vi "Lab Panel V4.87.vi"() -> ()   [LabVIEW 2013] (continued)
                    n2528 = call "sub vi - cycle&temp fail v6.vi"("Amps Lo?"=w4753, "Input Cluster"=w4741, "SELECT"=w4750, "Amps Hi?"=w4749, "Result In"=w4743) -> ("(FAIL) out"=w4745:cluster{"FAIL LO":dbl, "FAIL HI":dbl}, "(DISP) out"=w4748:T4, "T-RISE"=w4742:cluster{"T-RISE (L)":dbl, "T-RISE (N)":dbl}, "Result Out"=w4744:bool, "file error"=w4747:errorcluster)  [unwired: 10 in]
                    n2529 = local write "FAIL LAB03-2"(w4745) -> ()
                    n2530 = local write "TEMP RISE LAB03-2"(w4742) -> ()
                    n2531 = local write "DISP LAB03-2"(w4748) -> ()
                    n2532 = local write "RESULT LAB03-2"(w4744) -> ()
                    n2533 = local write "data file error"(w4747) -> ()
                  }
                }
              }
              frame #6 {
                # "LAB04-1"
                n2534 = case shown="True" w4758 {
                  tunnel: w4760 -> [_ w4773]
                  tunnel: w4757 -> [_ w4770]
                  tunnel: w4759 -> [_ w4769]
                  frame False {
                  }
                  frame True {
                    n2535 = local read "TEMP START LAB04-1"() -> (w4775:cluster{"TL":dbl, "TN":dbl})
                    n2536 = local read "FAIL LAB04-1"() -> (w4766:cluster{"LO":dbl, "HI":dbl})
                    n2537 = local read "TDMS LAB04-1"() -> (w4774:refnum<k34>)
                    n2538 = local read "SET LAB04-1"() -> (w4771:T5)
                    n2539 = local read "DISP LAB04-1"() -> (w4772:T4)
                    n2540 = local read "SIG LAB04-1"() -> (w4776:T2)
                    n2541 = local read "RESULT LAB04-1"() -> (w4763:bool)
                    n2542 = Bundle("FAIL LAB04-1"=w4766, "SIG LAB04-1"=w4776, "TEMP START LAB04-1"=w4775, "DISP LAB04-1"=w4772, "SET LAB04-1"=w4771, "TDMS LAB04-1"=w4774) -> (w4761:T38)  [unwired: 1 in]
                    n2543 = call "sub vi - cycle&temp fail v6.vi"("Amps Lo?"=w4773, "Input Cluster"=w4761, "SELECT"=w4770, "Amps Hi?"=w4769, "Result In"=w4763) -> ("(FAIL) out"=w4765:cluster{"FAIL LO":dbl, "FAIL HI":dbl}, "(DISP) out"=w4768:T4, "T-RISE"=w4762:cluster{"T-RISE (L)":dbl, "T-RISE (N)":dbl}, "Result Out"=w4764:bool, "file error"=w4767:errorcluster)  [unwired: 10 in]
                    n2544 = local write "TEMP RISE LAB04-1"(w4762) -> ()
                    n2545 = local write "FAIL LAB04-1"(w4765) -> ()
                    n2546 = local write "DISP LAB04-1"(w4768) -> ()
                    n2547 = local write "RESULT LAB04-1"(w4764) -> ()
                    n2548 = local write "data file error"(w4767) -> ()
                  }
                }
              }
              frame #7 {
                # "LAB04-2"
                n2549 = case shown="True" w4778 {
                  tunnel: w4780 -> [_ w4793]
                  tunnel: w4777 -> [_ w4790]
                  tunnel: w4779 -> [_ w4789]
                  frame False {
                  }
                  frame True {
                    n2550 = local read "TEMP START LAB04-2"() -> (w4795:cluster{"TL":dbl, "TN":dbl})
                    n2551 = local read "FAIL LAB04-2"() -> (w4786:cluster{"LO":dbl, "HI":dbl})
                    n2552 = local read "TDMS LAB04-2"() -> (w4794:refnum<k34>)
                    n2553 = local read "SET LAB04-2"() -> (w4791:T5)
                    n2554 = local read "DISP LAB04-2"() -> (w4792:T4)
                    n2555 = local read "SIG LAB04-2"() -> (w4796:T2)
                    n2556 = local read "RESULT LAB04-2"() -> (w4783:bool)
                    n2557 = Bundle("FAIL LAB04-2"=w4786, "SIG LAB04-2"=w4796, "TEMP START LAB04-2"=w4795, "DISP LAB04-2"=w4792, "SET LAB04-2"=w4791, "TDMS LAB04-2"=w4794) -> (w4781:T39)  [unwired: 1 in]
                    n2558 = call "sub vi - cycle&temp fail v6.vi"("Amps Lo?"=w4793, "Input Cluster"=w4781, "SELECT"=w4790, "Amps Hi?"=w4789, "Result In"=w4783) -> ("(FAIL) out"=w4785:cluster{"FAIL LO":dbl, "FAIL HI":dbl}, "(DISP) out"=w4788:T4, "T-RISE"=w4782:cluster{"T-RISE (L)":dbl, "T-RISE (N)":dbl}, "Result Out"=w4784:bool, "file error"=w4787:errorcluster)  [unwired: 10 in]
                    n2559 = local write "TEMP RISE LAB04-2"(w4782) -> ()
                    n2560 = local write "FAIL LAB04-2"(w4785) -> ()
                    n2561 = local write "DISP LAB04-2"(w4788) -> ()
                    n2562 = local write "RESULT LAB04-2"(w4784) -> ()
                    n2563 = local write "data file error"(w4787) -> ()
                  }
                }
              }
              frame #8 {
                # "LAB05-1"
                n2564 = case shown="True" w4798 {
                  tunnel: w4800 -> [_ w4813]
                  tunnel: w4797 -> [_ w4810]
                  tunnel: w4799 -> [_ w4809]
                  frame False {
                  }
                  frame True {
                    n2565 = local read "TEMP START LAB05-1"() -> (w4815:cluster{"TL":dbl, "TN":dbl})
                    n2566 = local read "FAIL LAB05-1"() -> (w4806:cluster{"LO":dbl, "HI":dbl})
                    n2567 = local read "TDMS LAB05-1"() -> (w4814:refnum<k34>)
                    n2568 = local read "SET LAB05-1"() -> (w4811:T5)
                    n2569 = local read "DISP LAB05-1"() -> (w4812:T4)
                    n2570 = local read "SIG LAB05-1"() -> (w4816:T2)
                    n2571 = local read "RESULT LAB05-1"() -> (w4803:bool)
                    n2572 = Bundle("FAIL LAB05-1"=w4806, "SIG LAB05-1"=w4816, "TEMP START LAB05-1"=w4815, "DISP LAB05-1"=w4812, "SET LAB05-1"=w4811, "TDMS LAB05-1"=w4814) -> (w4801:T40)  [unwired: 1 in]
                    n2573 = call "sub vi - cycle&temp fail v6.vi"("Amps Lo?"=w4813, "Input Cluster"=w4801, "SELECT"=w4810, "Amps Hi?"=w4809, "Result In"=w4803) -> ("(FAIL) out"=w4805:cluster{"FAIL LO":dbl, "FAIL HI":dbl}, "(DISP) out"=w4808:T4, "T-RISE"=w4802:cluster{"T-RISE (L)":dbl, "T-RISE (N)":dbl}, "Result Out"=w4804:bool, "file error"=w4807:errorcluster)  [unwired: 10 in]
                    n2574 = local write "TEMP RISE LAB05-1"(w4802) -> ()
                    n2575 = local write "FAIL LAB05-1"(w4805) -> ()
                    n2576 = local write "DISP LAB05-1"(w4808) -> ()
                    n2577 = local write "RESULT LAB05-1"(w4804) -> ()
                    n2578 = local write "data file error"(w4807) -> ()
                  }
                }
              }
              frame #9 {
                # "LAB05-2"
                n2579 = case shown="True" w4818 {
                  tunnel: w4820 -> [_ w4833]
                  tunnel: w4817 -> [_ w4830]
                  tunnel: w4819 -> [_ w4829]
                  frame False {
                  }
                  frame True {
                    n2580 = local read "TEMP START LAB05-2"() -> (w4835:cluster{"TL":dbl, "TN":dbl})
                    n2581 = local read "FAIL LAB05-2"() -> (w4826:cluster{"LO":dbl, "HI":dbl})
                    n2582 = local read "TDMS LAB05-2"() -> (w4834:refnum<k34>)
                    n2583 = local read "SET LAB05-2"() -> (w4831:T5)
                    n2584 = local read "DISP LAB05-2"() -> (w4832:T4)
                    n2585 = local read "SIG LAB05-2"() -> (w4836:T2)
                    n2586 = local read "RESULT LAB05-2"() -> (w4823:bool)
                    n2587 = Bundle("FAIL LAB05-2"=w4826, "SIG LAB05-2"=w4836, "TEMP START LAB05-2"=w4835, "DISP LAB05-2"=w4832, "SET LAB05-2"=w4831, "TDMS LAB05-2"=w4834) -> (w4821:T41)  [unwired: 1 in]
                    n2588 = call "sub vi - cycle&temp fail v6.vi"("Amps Lo?"=w4833, "Input Cluster"=w4821, "SELECT"=w4830, "Amps Hi?"=w4829, "Result In"=w4823) -> ("(FAIL) out"=w4825:cluster{"FAIL LO":dbl, "FAIL HI":dbl}, "(DISP) out"=w4828:T4, "T-RISE"=w4822:cluster{"T-RISE (L)":dbl, "T-RISE (N)":dbl}, "Result Out"=w4824:bool, "file error"=w4827:errorcluster)  [unwired: 10 in]
                    n2589 = local write "TEMP RISE LAB05-2"(w4822) -> ()
                    n2590 = local write "FAIL LAB05-2"(w4825) -> ()
                    n2591 = local write "DISP LAB05-2"(w4828) -> ()
                    n2592 = local write "RESULT LAB05-2"(w4824) -> ()
                    n2593 = local write "data file error"(w4827) -> ()
                  }
                }
              }
            }
          }
          frame #15 {
            # "run calibration routine"
            n2594 = local read "SET (cal)"() -> (w4837:bool)
            n2595 = case shown="True" w4837 {
              frame False {
              }
              frame True {
                n2596 = stacked-sequence {
                  seq-local: [w4838 _ _] -> [_ w4840 _]
                  frame #0 {
                    n2597 = call "CALIBRATION PASSWORD"() -> ("PASSWORD"=w4838:string)  [unwired: 17 in, 2 out]
                  }
                  frame #1 {
                    n2598 = Equal?(x=w4840, y="7777") -> (x = y?=w4839:bool)
                    n2599 = case shown="True" w4839 {
                      frame False {
                      }
                      frame True {
                        n2600 = stacked-sequence {
                          frame #0 {
                            n2601 = call "sub vi - calibration v1.vi"() -> ()  [unwired: 12 in]
                          }
                          frame #1 {
                            n2602 = call "sub vi - get calibration values v1.vi"() -> ("LAB01 (CAL)"=w4846:T14, "LAB02 (CAL)"=w4845:T15, "LAB03 (CAL)"=w4844:T14, "LAB04 (CAL)"=w4843:T14, "calibration file error out"=w4847:errorcluster, "LAB05 (CAL)"=w4842:T14)  [unwired: 9 in, 1 out]
                            n2603 = local write "cal file error out"(w4847) -> ()
                            n2604 = local write "CAL LAB04"(w4843) -> ()
                            n2605 = local write "CAL LAB05"(w4842) -> ()
                            n2606 = local write "CAL LAB01"(w4846) -> ()
                            n2607 = local write "CAL LAB02"(w4845) -> ()
                            n2608 = local write "CAL LAB03"(w4844) -> ()
                          }
                        }
                      }
                    }
                  }
                  frame #2 {
                    n2609 = local write "SET (cal)"(FALSE) -> ()
                  }
                }
              }
            }
          }
          frame #16 {
            # "save certain settings to file"
            n2610 = String To Path(string="c:\\crabtree\\Set Up\\") -> (path=w4850:path)
            n2611 = Build Path(base path=w4850, name or relative path="settings.bin") -> (appended path=w4852:path)
            n2612 = Build Path(base path=w4850, name or relative path="mail.bin") -> (appended path=w4849:path)
            n2613 = Create Folder(path (use dialog)=w4850) -> (error out=w4855:errorcluster)  [unwired: 2 in, 2 out]
            n2614 = call <vilib>:"Clear Errors.vi"("error in (no error)"=w4855) -> ()  [unwired: 6 in, 1 out]
            n2615 = stacked-sequence {
              seq-local: [w4867 _] -> [_ w4880]
              tunnel: w4852 -> [_ w4881]
              tunnel: w4849 -> [_ w4879]
              frame #0 {
                n2616 = local read "C drive data root dir"() -> (w4866:path)
                n2617 = local read "Select COM port"() -> (w4863:refnum<visa-resource-name>)
                n2618 = local read "Network Directory"() -> (w4872:path)
                n2619 = local read "SET LAB05-2"() -> (w4871:T5)
                n2620 = local read "SET LAB05-1"() -> (w4870:T5)
                n2621 = local read "SET LAB04-2"() -> (w4869:T5)
                n2622 = local read "SET LAB03-2"() -> (w4873:T5)
                n2623 = local read "SET LAB04-1"() -> (w4868:T5)
                n2624 = local read "SET LAB03-1"() -> (w4874:T5)
                n2625 = local read "SET LAB02-2"() -> (w4875:T5)
                n2626 = local read "SET LAB02-1"() -> (w4876:T5)
                n2627 = local read "Temp Delay Lps"() -> (w4862:dbl)
                n2628 = local read "SET LAB01-2"() -> (w4877:T5)
                n2629 = local read "Temp Test Cal"() -> (w4859:dbl)
                n2630 = local read "SET LAB01-1"() -> (w4878:T5)
                n2631 = local read "Mail Test File To:"() -> (w4857:string)
                n2632 = local read "Temp Value"() -> (w4861:dbl)
                n2633 = local read "Fail Loops"() -> (w4860:dbl)
                n2634 = local read "spare"() -> (w4858:dbl)
                n2635 = local read "Mail Test Fail"() -> (w4856:bool)
                n2636 = local read "RATE (Hz)"() -> (w4865:dbl)
                n2637 = local read "SAMPLES"() -> (w4864:dbl)
                n2638 = Bundle("SET LAB01-1"=w4878, "SET LAB01-2"=w4877, "SET LAB02-1"=w4876, "SET LAB02-2"=w4875, "SET LAB03-1"=w4874, "SET LAB03-2"=w4873, "SET LAB04-1"=w4868, "SET LAB04-2"=w4869, "SET LAB05-1"=w4870, "SET LAB05-2"=w4871, "Network Directory"=w4872, "C drive data root dir"=w4866, "RATE (Hz)"=w4865, "SAMPLES"=w4864, "Select COM port"=w4863, "Temp Delay Lps"=w4862, "Temp Value"=w4861, "Fail Loops"=w4860, "Temp Test Cal"=w4859, "spare"=w4858, "Mail Test File To:"=w4857, "Mail Test Fail"=w4856) -> (w4867:T22)  [unwired: 1 in]
              }
              frame #1 {
                n2639 = event shown="[1] \"SET LAB01-1\", \"SET LAB01-2\", \"SET LAB02-1\", \"SET LAB02-2\", \"SET LAB03-1\", \"SET LAB03-2\", \"SET LAB04-1\", \"SET LAB04-2\", \"SET LAB05-1\", \"SET LAB05-2\", \"Network Directory\", \"C drive data root dir\", \"RATE (Hz)\", \"SAMPLES\", \"Select COM port\", \"Temp Delay Lps\", \"Temp Value\", \"Fail Loops\", \"Temp Test Cal\", \"spare\", \"Mail Test File To:\", \"Mail Test Fail\": Value Change" {
                  selector: _ -> [_ _ _]
                  dyn-events: _ -> [_ _ _]
                  timeout: 10.0 -> [_ _ _]
                  tunnel: w4881 -> [_ w4883 _]
                  tunnel: w4880 -> [_ w4884 _]
                  tunnel: w4879 -> [_ _ w4895]
                  event Timeout {
                    n2640 = event-data() -> ()  [unwired: 1 in, 3 out]
                  }
                  event "SET LAB01-1", "SET LAB01-2", "SET LAB02-1", "SET LAB02-2", "SET LAB03-1", "SET LAB03-2", "SET LAB04-1", "SET LAB04-2", "SET LAB05-1", "SET LAB05-2", "Network Directory", "C drive data root dir", "RATE (Hz)", "SAMPLES", "Select COM port", "Temp Delay Lps", "Temp Value", "Fail Loops", "Temp Test Cal", "spare", "Mail Test File To:", "Mail Test Fail": Value Change {
                    n2641 = event-data() -> ()  [unwired: 1 in, 6 out]
                    n2642 = Open/Create/Replace File(file path (use dialog)=w4883, operation (0:open)=T21."replace or create") -> (refnum out=w4889:refnum<file>, error out=w4888:errorcluster)  [unwired: 4 in, 1 out]
                    n2643 = Write to Binary File(file (use dialog)=w4889, data=w4884, error in=w4888) -> (refnum out=w4887:refnum<file>, error out=w4886:errorcluster)  [unwired: 3 in, 1 out]
                    n2644 = Close File(refnum=w4887, error in=w4886) -> (error out=w4885:errorcluster)  [unwired: 1 out]
                    n2645 = local write "data file error"(w4885) -> ()
                  }
                  event "MAIL SETTINGS.OUT SERVER ADDRESS", "MAIL SETTINGS.FROM ACCOUNT", "MAIL SETTINGS.USER NAME", "MAIL SETTINGS.PASSWORD", "Auto Mail Send", "TO (string):": Value Change {
                    n2646 = event-data() -> ()  [unwired: 1 in, 6 out]
                    n2647 = local read "MAIL SETTINGS"() -> (w4894:T7)
                    n2648 = local read "Auto Mail Send"() -> (w4892:bool)
                    n2649 = local read "TO (string):"() -> (w4891:string)
                    n2650 = Open/Create/Replace File(file path (use dialog)=w4895, operation (0:open)=T21."replace or create") -> (refnum out=w4900:refnum<file>, error out=w4899:errorcluster)  [unwired: 4 in, 1 out]
                    n2651 = Bundle("MAIL SETTINGS"=w4894, "Auto Mail Send"=w4892, "TO (string):"=w4891) -> (w4893:T42)  [unwired: 1 in]
                    n2652 = Write to Binary File(file (use dialog)=w4900, data=w4893, error in=w4899) -> (refnum out=w4898:refnum<file>, error out=w4897:errorcluster)  [unwired: 3 in, 1 out]
                    n2653 = Close File(refnum=w4898, error in=w4897) -> (error out=w4896:errorcluster)  [unwired: 1 out]
                    n2654 = local write "data file error"(w4896) -> ()
                  }
                }
              }
            }
          }
          frame #17 {
            # "mail control"
            n2655 = local read "MAIL SETTINGS"() -> (w4917:T7)
            n2656 = local read "Auto Mail Send"() -> (w4903:bool)
            n2657 = Unbundle(w4917) -> ("OUT SERVER ADDRESS"=w4916:string, "FROM ACCOUNT"=w4915:string, "TEST MAIL"=w4914:bool)  [unwired: 4 out]
            n2658 = stacked-sequence {
              tunnel: "TO (string):" -> [_ w4956]
              tunnel: w4917 -> [w4922 w4955]
              tunnel: w4916 -> [w4921 w4954]
              tunnel: w4915 -> [w4920 w4953]
              tunnel: w4914 -> [w4919 _]
              tunnel: w4903 -> [_ w4952]
              tunnel: w4913 -> [_ w4951]
              tunnel: w4912 -> [_ w4950]
              tunnel: w4911 -> [_ w4949]
              tunnel: w4910 -> [_ w4948]
              tunnel: w4909 -> [_ w4947]
              tunnel: w4908 -> [_ w4946]
              tunnel: w4907 -> [_ w4945]
              tunnel: w4906 -> [_ w4944]
              tunnel: w4905 -> [_ w4943]
              tunnel: w4904 -> [_ w4942]
              tunnel: "TO (string):" -> [w4918 _]
              frame #0 {
                # "mail test"
                n2659 = case shown="True" w4919 {
                  tunnel: w4922 -> [_ w4926]
                  tunnel: w4918 -> [_ w4925]
                  tunnel: w4921 -> [_ w4924]
                  tunnel: w4920 -> [_ w4923]
                  frame False {
                  }
                  frame True {
                    n2660 = stacked-sequence {
                      seq-local: [_ _ w4936 _] -> [_ _ _ w4937]
                      tunnel: w4926 -> [w4929 _ _ w4941]
                      tunnel: w4925 -> [_ _ w4934 _]
                      tunnel: w4924 -> [_ _ w4932 _]
                      tunnel: w4923 -> [_ _ w4933 _]
                      frame #0 {
                        n2661 = Bundle(cluster=w4929, "TEST MAIL STATUS"="TEST START") -> (w4927:T7)  [unwired: 6 in]
                        n2662 = local write "MAIL SETTINGS"(w4927) -> ()
                      }
                      frame #1 {
                        n2663 = Wait (ms)(milliseconds to wait=500) -> ()  [unwired: 1 out]
                      }
                      frame #2 {
                        n2664 = call "sub vi - send mail v5.vi"("TO:"=w4934, "subject"="MAIL TEST FROM LAB PANEL", "from"=w4933, "out going server"=w4932, "message"="TEST MESSAGE") -> ("error out"=w4936:errorcluster)  [unwired: 10 in]
                      }
                      frame #3 {
                        n2665 = Bundle(cluster=w4941, "TEST MAIL"=FALSE, "TEST MAIL STATUS"="TEST END", "mail error"=w4937) -> (w4939:T7)  [unwired: 4 in]
                        n2666 = local write "MAIL SETTINGS"(w4939) -> ()
                      }
                    }
                  }
                }
              }
              frame #1 {
                # "mail report"
                n2667 = stacked-sequence {
                  seq-local: [_ w4999 _ _] -> [_ _ _ w5189]
                  seq-local: [_ _ w5102 _] -> [_ _ _ w5179]
                  seq-local: [w4966 _ _ _] -> [_ w5016 _ _]
                  seq-local: [w4965 _ _ _] -> [_ w5015 _ _]
                  seq-local: [w4963 _ _ _] -> [_ w5013 _ _]
                  seq-local: [w4964 _ _ _] -> [_ w5014 _ _]
                  seq-local: [w4962 _ _ _] -> [_ w5012 _ _]
                  seq-local: [w4961 _ _ _] -> [_ w5007 _ _]
                  seq-local: [w4960 _ _ _] -> [_ w5008 _ _]
                  seq-local: [w4959 _ _ _] -> [_ w5009 _ _]
                  seq-local: [w4958 _ _ _] -> [_ w5010 _ _]
                  seq-local: [w4957 _ _ _] -> [_ w5011 _ _]
                  tunnel: w4956 -> [_ _ _ w5190]
                  tunnel: w4955 -> [_ _ _ w5173]
                  tunnel: w4954 -> [_ _ _ w5187]
                  tunnel: w4953 -> [_ _ _ w5186]
                  tunnel: w4952 -> [w4997 _ _ w5181]
                  tunnel: w4951 -> [_ _ w5132 _]
                  tunnel: w4950 -> [_ _ w5129 _]
                  tunnel: w4949 -> [_ _ w5128 _]
                  tunnel: w4948 -> [_ _ w5127 _]
                  tunnel: w4947 -> [_ _ w5126 _]
                  tunnel: w4946 -> [_ _ w5125 _]
                  tunnel: w4945 -> [_ _ w5124 _]
                  tunnel: w4944 -> [_ _ w5123 _]
                  tunnel: w4943 -> [_ _ w5122 _]
                  tunnel: w4942 -> [_ _ w5121 _]
                  frame #0 {
                    n2668 = case shown="False" w4997 {
                      frame False {
                        n2669 = local write "mail control"("") -> ()
                      }
                      frame True {
                      }
                    }
                    n2670 = local read "SET LAB01-1"() -> (w4996:T5)
                    n2671 = local read "SET LAB01-2"() -> (w4995:T5)
                    n2672 = local read "SET LAB02-1"() -> (w4994:T5)
                    n2673 = local read "SET LAB02-2"() -> (w4993:T5)
                    n2674 = local read "SET LAB03-1"() -> (w4992:T5)
                    n2675 = local read "SET LAB04-1"() -> (w4990:T5)
                    n2676 = local read "SET LAB05-1"() -> (w4988:T5)
                    n2677 = local read "SET LAB03-2"() -> (w4991:T5)
                    n2678 = local read "SET LAB04-2"() -> (w4989:T5)
                    n2679 = local read "SET LAB05-2"() -> (w4987:T5)
                    n2680 = Unbundle(w4992) -> ("DESCRIPTION"=w4972:string)  [unwired: 4 out]
                    n2681 = Unbundle(w4991) -> ("DESCRIPTION"=w4971:string)  [unwired: 4 out]
                    n2682 = Unbundle(w4990) -> ("DESCRIPTION"=w4970:string)  [unwired: 4 out]
                    n2683 = Unbundle(w4987) -> ("DESCRIPTION"=w4967:string)  [unwired: 4 out]
                    n2684 = Unbundle(w4993) -> ("DESCRIPTION"=w4973:string)  [unwired: 4 out]
                    n2685 = Unbundle(w4989) -> ("DESCRIPTION"=w4969:string)  [unwired: 4 out]
                    n2686 = Unbundle(w4996) -> ("DESCRIPTION"=w4985:string)  [unwired: 4 out]
                    n2687 = Unbundle(w4994) -> ("DESCRIPTION"=w4974:string)  [unwired: 4 out]
                    n2688 = Unbundle(w4988) -> ("DESCRIPTION"=w4968:string)  [unwired: 4 out]
                    n2689 = Unbundle(w4995) -> ("DESCRIPTION"=w4975:string)  [unwired: 4 out]
                    n2690 = Concatenate Strings("[LAB05-2/", w4967) -> (w4957:string)
                    n2691 = Concatenate Strings("[LAB05-1/", w4968) -> (w4958:string)
                    n2692 = Concatenate Strings("[LAB04-2/", w4969) -> (w4959:string)
                    n2693 = Concatenate Strings("[LAB03-2/", w4971) -> (w4961:string)
                    n2694 = Concatenate Strings("[LAB04-1/", w4970) -> (w4960:string)
                    n2695 = Concatenate Strings("[LAB03-1/", w4972) -> (w4962:string)
                    n2696 = Concatenate Strings("[LAB01-2/", w4975) -> (w4965:string)
                    n2697 = Concatenate Strings("[LAB02-2/", w4973) -> (w4963:string)
                    n2698 = Concatenate Strings("[LAB01-1/", w4985) -> (w4966:string)
                    n2699 = Concatenate Strings("[LAB02-1/", w4974) -> (w4964:string)
                  }
                  frame #1 {
                    w5020 = "/"
                    w5021 = 2.0
                    n2700 = local read "DISP LAB01-2"() -> (w5100:T4)
                    n2701 = local read "DISP LAB01-1"() -> (w5101:T4)
                    n2702 = local read "DISP LAB02-1"() -> (w5099:T4)
                    n2703 = local read "DISP LAB03-2"() -> (w5096:T4)
                    n2704 = local read "DISP LAB02-2"() -> (w5098:T4)
                    n2705 = local read "DISP LAB03-1"() -> (w5097:T4)
                    n2706 = local read "DISP LAB04-2"() -> (w5094:T4)
                    n2707 = local read "DISP LAB04-1"() -> (w5095:T4)
                    n2708 = local read "DISP LAB05-1"() -> (w5093:T4)
                    n2709 = local read "DISP LAB05-2"() -> (w5092:T4)
                    n2710 = Unbundle(w5100) -> ("CYCLE"=w5084:dbl, "MINS"=w5083:dbl, "STATUS"=w5080:string)
                    n2711 = Unbundle(w5101) -> ("CYCLE"=w5089:dbl, "MINS"=w5088:dbl, "STATUS"=w5085:string)
                    n2712 = Unbundle(w5099) -> ("CYCLE"=w5077:dbl, "MINS"=w5076:dbl, "STATUS"=w5075:string)
                    n2713 = Unbundle(w5096) -> ("CYCLE"=w5064:dbl, "MINS"=w5063:dbl, "STATUS"=w5060:string)
                    n2714 = Unbundle(w5097) -> ("CYCLE"=w5069:dbl, "MINS"=w5068:dbl, "STATUS"=w5065:string)
                    n2715 = Unbundle(w5098) -> ("CYCLE"=w5074:dbl, "MINS"=w5073:dbl, "STATUS"=w5070:string)
                    n2716 = Unbundle(w5095) -> ("CYCLE"=w5059:dbl, "MINS"=w5058:dbl, "STATUS"=w5055:string)
                    n2717 = Unbundle(w5094) -> ("CYCLE"=w5054:dbl, "MINS"=w5053:dbl, "STATUS"=w5050:string)
                    n2718 = Unbundle(w5093) -> ("CYCLE"=w5049:dbl, "MINS"=w5048:dbl, "STATUS"=w5045:string)
                    n2719 = Unbundle(w5092) -> ("CYCLE"=w5091:dbl, "MINS"=w5090:dbl, "STATUS"=w5042:string)
                    n2720 = Number To Decimal String(number=w5077) -> (decimal integer string=w5079:string)  [unwired: 1 in]
                    n2721 = Number To Decimal String(number=w5074) -> (decimal integer string=w5072:string)  [unwired: 1 in]
                    n2722 = Number To Decimal String(number=w5069) -> (decimal integer string=w5067:string)  [unwired: 1 in]
                    n2723 = Number To Decimal String(number=w5084) -> (decimal integer string=w5082:string)  [unwired: 1 in]
                    n2724 = Number To Decimal String(number=w5064) -> (decimal integer string=w5062:string)  [unwired: 1 in]
                    n2725 = Number To Decimal String(number=w5089) -> (decimal integer string=w5087:string)  [unwired: 1 in]
                    n2726 = Number To Decimal String(number=w5091) -> (decimal integer string=w5044:string)  [unwired: 1 in]
                    n2727 = Number To Decimal String(number=w5059) -> (decimal integer string=w5057:string)  [unwired: 1 in]
                    n2728 = Number To Decimal String(number=w5054) -> (decimal integer string=w5052:string)  [unwired: 1 in]
                    n2729 = Number To Decimal String(number=w5049) -> (decimal integer string=w5047:string)  [unwired: 1 in]
                    n2730 = Number To Fractional String(number=w5076, precision (6)=w5021) -> (F-format string=w5078:string)  [unwired: 2 in]
                    n2731 = Number To Fractional String(number=w5063, precision (6)=w5021) -> (F-format string=w5061:string)  [unwired: 2 in]
                    n2732 = Number To Fractional String(number=w5073, precision (6)=w5021) -> (F-format string=w5071:string)  [unwired: 2 in]
                    n2733 = Number To Fractional String(number=w5068, precision (6)=w5021) -> (F-format string=w5066:string)  [unwired: 2 in]
                    n2734 = Number To Fractional String(number=w5053, precision (6)=w5021) -> (F-format string=w5051:string)  [unwired: 2 in]
                    n2735 = Number To Fractional String(number=w5058, precision (6)=w5021) -> (F-format string=w5056:string)  [unwired: 2 in]
                    n2736 = Number To Fractional String(number=w5083, precision (6)=w5021) -> (F-format string=w5081:string)  [unwired: 2 in]
                    n2737 = Number To Fractional String(number=w5048, precision (6)=w5021) -> (F-format string=w5046:string)  [unwired: 2 in]
                    n2738 = Number To Fractional String(number=w5088, precision (6)=w5021) -> (F-format string=w5086:string)  [unwired: 2 in]
                    n2739 = Number To Fractional String(number=w5090, precision (6)=w5021) -> (F-format string=w5043:string)  [unwired: 2 in]
                    n2740 = Concatenate Strings(w5020, w5062, w5020, w5061, w5020, w5060) -> (w5036:string)
                    n2741 = Concatenate Strings(w5020, w5057, w5020, w5056, w5020, w5055) -> (w5035:string)
                    n2742 = Concatenate Strings(w5020, w5052, w5020, w5051, w5020, w5050) -> (w5034:string)
                    n2743 = Concatenate Strings(w5020, w5047, w5020, w5046, w5020, w5045) -> (w5033:string)
                    n2744 = Concatenate Strings(w5020, w5044, w5020, w5043, w5020, w5042) -> (w5032:string)
                    n2745 = Concatenate Strings(w5020, w5087, w5020, w5086, w5020, w5085) -> (w5041:string)
                    n2746 = Concatenate Strings(w5020, w5067, w5020, w5066, w5020, w5065) -> (w5037:string)
                    n2747 = Concatenate Strings(w5020, w5082, w5020, w5081, w5020, w5080) -> (w5040:string)
                    n2748 = Concatenate Strings(w5020, w5079, w5020, w5078, w5020, w5075) -> (w5039:string)
                    n2749 = Concatenate Strings(w5020, w5072, w5020, w5071, w5020, w5070) -> (w5038:string)
                    n2750 = Concatenate Strings("]", "\r") -> (w5017:string)
                    n2751 = Concatenate Strings(w5012, w5037, w5017) -> (w5027:string)
                    n2752 = Concatenate Strings(w5014, w5039, w5017) -> (w5029:string)
                    n2753 = Concatenate Strings(w5013, w5038, w5017) -> (w5028:string)
                    n2754 = Concatenate Strings(w5009, w5034, w5017) -> (w5024:string)
                    n2755 = Concatenate Strings(w5010, w5033, w5017) -> (w5025:string)
                    n2756 = Concatenate Strings(w5008, w5035, w5017) -> (w5023:string)
                    n2757 = Concatenate Strings(w5007, w5036, w5017) -> (w5022:string)
                    n2758 = Concatenate Strings(w5011, w5032, w5017) -> (w5026:string)
                    n2759 = Concatenate Strings(w5015, w5040, w5017) -> (w5030:string)
                    n2760 = Concatenate Strings(w5016, w5041, w5017) -> (w5031:string)
                    n2761 = Concatenate Strings(w5031, w5030, w5029, w5028, w5027, w5022, w5023, w5024, w5025, w5026) -> (w5000:string)
                    n2762 = Concatenate Strings("[PANEL/", "DESC/", "CYCLES/", "MINS/", "STATUS]", "\r", w5000) -> (w4999:string)
                    "MAIL REPORT" <- w4999
                    n2763 = global write "Global display 3.vi" "log all"(w4999) -> ()
                  }
                  frame #2 {
                    w5130 = "END"
                    n2764 = local read "mail control"() -> (w5131:string)
                    n2765 = case shown="False" w5126 {
                      tunnel: w5131 -> [w5155 _]
                      tunnel: w5130 -> [w5154 _]
                      tunnel: [w5153 FALSE] -> w5116
                      frame False {
                        n2766 = Equal?(x=w5155, y=w5154) -> (x = y?=w5153:bool)
                      }
                      frame True {
                      }
                    }
                    n2767 = case shown="False" w5132 {
                      tunnel: w5131 -> [w5171 _]
                      tunnel: w5130 -> [w5170 _]
                      tunnel: [w5169 FALSE] -> w5120
                      frame False {
                        n2768 = Equal?(x=w5171, y=w5170) -> (x = y?=w5169:bool)
                      }
                      frame True {
                      }
                    }
                    n2769 = case shown="False" w5129 {
                      tunnel: w5131 -> [w5167 _]
                      tunnel: w5130 -> [w5166 _]
                      tunnel: [w5165 FALSE] -> w5119
                      frame False {
                        n2770 = Equal?(x=w5167, y=w5166) -> (x = y?=w5165:bool)
                      }
                      frame True {
                      }
                    }
                    n2771 = case shown="False" w5127 {
                      tunnel: w5131 -> [w5159 _]
                      tunnel: w5130 -> [w5158 _]
                      tunnel: [w5157 FALSE] -> w5117
                      frame False {
                        n2772 = Equal?(x=w5159, y=w5158) -> (x = y?=w5157:bool)
                      }
                      frame True {
                      }
                    }
                    n2773 = case shown="False" w5128 {
                      tunnel: w5131 -> [w5163 _]
                      tunnel: w5130 -> [w5162 _]
                      tunnel: [w5161 FALSE] -> w5118
                      frame False {
                        n2774 = Equal?(x=w5163, y=w5162) -> (x = y?=w5161:bool)
                      }
                      frame True {
                      }
                    }
                    n2775 = Or(x=w5118, y=w5117) -> (x .or. y?=w5109:bool)
                    n2776 = Or(x=w5120, y=w5119) -> (x .or. y?=w5110:bool)
                    n2777 = Or(x=w5110, y=w5109) -> (x .or. y?=w5105:bool)
                    n2778 = case shown="False" w5122 {
                      tunnel: w5131 -> [w5139 _]
                      tunnel: w5130 -> [w5138 _]
                      tunnel: [w5137 FALSE] -> w5111
                      frame False {
                        n2779 = Equal?(x=w5139, y=w5138) -> (x = y?=w5137:bool)
                      }
                      frame True {
                      }
                    }
                    n2780 = case shown="False" w5121 {
                      tunnel: w5131 -> [w5135 _]
                      tunnel: w5130 -> [w5134 _]
                      tunnel: [w5133 FALSE] -> w5115
                      frame False {
                        n2781 = Equal?(x=w5135, y=w5134) -> (x = y?=w5133:bool)
                      }
                      frame True {
                      }
                    }
                    n2782 = case shown="False" w5123 {
                      tunnel: w5131 -> [w5143 _]
                      tunnel: w5130 -> [w5142 _]
                      tunnel: [w5141 FALSE] -> w5112
                      frame False {
                        n2783 = Equal?(x=w5143, y=w5142) -> (x = y?=w5141:bool)
                      }
                      frame True {
                      }
                    }
                    n2784 = case shown="False" w5125 {
                      tunnel: w5131 -> [w5151 _]
                      tunnel: w5130 -> [w5150 _]
                      tunnel: [w5149 FALSE] -> w5114
                      frame False {
                        n2785 = Equal?(x=w5151, y=w5150) -> (x = y?=w5149:bool)
                      }
                      frame True {
                      }
                    }
                    n2786 = case shown="False" w5124 {
                      tunnel: w5131 -> [w5147 _]
                      tunnel: w5130 -> [w5146 _]
                      tunnel: [w5145 FALSE] -> w5113
                      frame False {
                        n2787 = Equal?(x=w5147, y=w5146) -> (x = y?=w5145:bool)
                      }
                      frame True {
                      }
                    }
                    n2788 = Or(x=w5114, y=w5113) -> (x .or. y?=w5108:bool)
                    n2789 = Or(x=w5112, y=w5111) -> (x .or. y?=w5107:bool)
                    n2790 = Or(x=w5115, y=w5116) -> (x .or. y?=w5103:bool)
                    n2791 = Or(x=w5108, y=w5107) -> (x .or. y?=w5106:bool)
                    n2792 = Or(x=w5105, y=w5106) -> (x .or. y?=w5104:bool)
                    n2793 = Or(x=w5104, y=w5103) -> (x .or. y?=w5102:bool)
                  }
                  frame #3 {
                    n2794 = local read "on loops"() -> (w5185:dbl)
                    n2795 = local read "jig cycle"() -> (w5182:dbl)
                    n2796 = local read "Send Mail Now"() -> (w5176:bool)
                    n2797 = Add(x=w5185, y=3.0) -> (x+y=w5183:dbl)
                    n2798 = Equal?(x=w5182, y=w5183) -> (x = y?=w5177:bool)
                    n2799 = And(x=w5177, y=w5176) -> (x .and. y?=w5175:bool)
                    n2800 = And(x=w5181, y=w5177) -> (x .and. y?=w5180:bool)
                    n2801 = And(x=w5180, y=w5179) -> (x .and. y?=w5178:bool)
                    n2802 = Or(x=w5178, y=w5175) -> (x .or. y?=w5174:bool)
                    n2803 = case shown="True" w5174 {
                      tunnel: w5190 -> [_ w5196]
                      tunnel: w5189 -> [_ w5195]
                      tunnel: "Lab Panel Test Status" -> [_ w5194]
                      tunnel: w5187 -> [_ w5193]
                      tunnel: w5186 -> [_ w5192]
                      tunnel: w5173 -> [_ w5191]
                      frame False {
                      }
                      frame True {
                        n2804 = stacked-sequence {
                          tunnel: w5196 -> [w5204 _]
                          tunnel: w5195 -> [w5203 _]
                          tunnel: w5194 -> [w5202 _]
                          tunnel: w5193 -> [w5201 _]
                          tunnel: w5192 -> [w5200 _]
                          tunnel: w5191 -> [w5199 _]
                          frame #0 {
                            n2805 = call "sub vi - send mail v5.vi"("TO:"=w5204, "subject"=w5202, "from"=w5200, "out going server"=w5201, "message"=w5203) -> ("error out"=w5198:errorcluster)  [unwired: 10 in]
                            n2806 = Bundle(cluster=w5199, "mail error"=w5198) -> (w5197:T7)  [unwired: 6 in]
                            n2807 = local write "MAIL SETTINGS"(w5197) -> ()
                          }
                          frame #1 {
                            n2808 = local write "mail control"("") -> ()
                            n2809 = local write "Send Mail Now"(FALSE) -> ()
                          }
                        }
                      }
                    }
                  }
                }
              }
            }
          }
          frame #18 {
            # "save jig cycle values once all run switches are off"
            n2810 = stacked-sequence {
              tunnel: w5216 -> [_ w5245]
              tunnel: w5215 -> [_ w5244]
              tunnel: w5214 -> [_ w5243]
              tunnel: w5213 -> [_ w5242]
              tunnel: w5212 -> [_ w5241]
              tunnel: w5211 -> [_ w5240]
              tunnel: w5210 -> [_ w5239]
              tunnel: w5209 -> [_ w5238]
              tunnel: w5208 -> [_ w5237]
              tunnel: w5207 -> [_ w5236]
              frame #0 {
              }
              frame #1 {
                n2811 = Not(x=w5236) -> (.not. x?=w5219:bool)
                n2812 = Not(x=w5244) -> (.not. x?=w5234:bool)
                n2813 = Not(x=w5241) -> (.not. x?=w5229:bool)
                n2814 = Not(x=w5239) -> (.not. x?=w5225:bool)
                n2815 = Not(x=w5237) -> (.not. x?=w5221:bool)
                n2816 = Not(x=w5245) -> (.not. x?=w5235:bool)
                n2817 = Not(x=w5243) -> (.not. x?=w5233:bool)
                n2818 = Not(x=w5240) -> (.not. x?=w5227:bool)
                n2819 = Not(x=w5242) -> (.not. x?=w5231:bool)
                n2820 = Not(x=w5238) -> (.not. x?=w5223:bool)
                n2821 = local read "Save JC"() -> (w5247:bool)
                n2822 = And(x=w5235, y=w5234) -> (x .and. y?=w5232:bool)
                n2823 = And(x=w5232, y=w5233) -> (x .and. y?=w5230:bool)
                n2824 = And(x=w5230, y=w5231) -> (x .and. y?=w5228:bool)
                n2825 = And(x=w5228, y=w5229) -> (x .and. y?=w5226:bool)
                n2826 = And(x=w5226, y=w5227) -> (x .and. y?=w5224:bool)
                n2827 = And(x=w5224, y=w5225) -> (x .and. y?=w5222:bool)
                n2828 = And(x=w5222, y=w5223) -> (x .and. y?=w5220:bool)
                n2829 = And(x=w5220, y=w5221) -> (x .and. y?=w5218:bool)
                n2830 = And(x=w5218, y=w5219) -> (x .and. y?=w5217:bool)
                n2831 = And(x=w5217, y=w5247) -> (x .and. y?=w5246:bool)
                n2832 = case shown="True" w5246 {
                  tunnel: w5217 -> [w5248 _]
                  frame False {
                    n2833 = case shown="False" w5248 {
                      frame False {
                        n2834 = local write "Save JC"(TRUE) -> ()
                      }
                      frame True {
                      }
                    }
                  }
                  frame True {
                    n2835 = stacked-sequence {
                      frame #0 {
                        n2836 = String To Path(string="c:\\crabtree\\Jig Cycles\\") -> (path=w5260:path)
                        n2837 = Build Path(base path=w5260, name or relative path="jigcycles.bin") -> (appended path=w5258:path)
                        n2838 = Create Folder(path (use dialog)=w5260) -> (error out=w5262:errorcluster)  [unwired: 2 in, 2 out]
                        n2839 = local read "JIG RELAY CYCLES"() -> (w5252:T8)
                        n2840 = call <vilib>:"Clear Errors.vi"("error in (no error)"=w5262) -> ()  [unwired: 6 in, 1 out]
                        n2841 = local write "Save JC"(FALSE) -> ()
                        n2842 = Open/Create/Replace File(file path (use dialog)=w5258, operation (0:open)=T21."replace or create") -> (refnum out=w5256:refnum<file>, error out=w5257:errorcluster)  [unwired: 4 in, 1 out]
                        n2843 = Write to Binary File(file (use dialog)=w5256, data=w5252, error in=w5257) -> (refnum out=w5255:refnum<file>, error out=w5254:errorcluster)  [unwired: 3 in, 1 out]
                        n2844 = Close File(refnum=w5255, error in=w5254) -> (error out=w5253:errorcluster)  [unwired: 1 out]
                        n2845 = local write "data file error"(w5253) -> ()
                      }
                      frame #1 {
                        n2846 = local read "JIG RELAY CYCLES"() -> (w5285:T8)
                        n2847 = Unbundle By Name(w5285) -> ("LAB01-1"=w5280:dbl, "LAB01-2"=w5279:dbl, "LAB02-1"=w5277:dbl, "LAB02-2"=w5276:dbl, "LAB03-1"=w5274:dbl, "LAB03-2"=w5271:dbl, "LAB04-1"=w5270:dbl, "LAB04-2"=w5268:dbl, "LAB05-1"=w5266:dbl, "LAB05-2"=w5264:dbl)
                        n2848 = stacked-sequence {
                          tunnel: w5280 -> [w5288 _ _ _ _ _ _ _ _ _]
                          tunnel: 1000000 -> [w5291 w5301 w5311 w5321 w5331 w5341 w5351 w5361 w5371 w5381]
                          tunnel: [w5289 _ _ _ _ _ _ _ _ _] -> w5283
                          tunnel: "TEST STATION HAS REACHED 1 MILLION CYCLES, REPLACE  CONTROL RELAYS" -> [w5287 w5299 w5309 w5319 w5329 w5339 w5349 w5359 w5369 w5379]
                          tunnel: [_ w5298 _ _ _ _ _ _ _ _] -> w5281
                          tunnel: w5279 -> [_ w5297 _ _ _ _ _ _ _ _]
                          tunnel: [_ _ w5308 _ _ _ _ _ _ _] -> w5278
                          tunnel: w5277 -> [_ _ w5307 _ _ _ _ _ _ _]
                          tunnel: w5276 -> [_ _ _ w5318 _ _ _ _ _ _]
                          tunnel: [_ _ _ w5317 _ _ _ _ _ _] -> w5275
                          tunnel: w5274 -> [_ _ _ _ w5328 _ _ _ _ _]
                          tunnel: [_ _ _ _ w5327 _ _ _ _ _] -> w5273
                          tunnel: [_ _ _ _ _ w5338 _ _ _ _] -> w5272
                          tunnel: w5271 -> [_ _ _ _ _ w5337 _ _ _ _]
                          tunnel: w5270 -> [_ _ _ _ _ _ w5348 _ _ _]
                          tunnel: [_ _ _ _ _ _ w5347 _ _ _] -> w5269
                          tunnel: w5268 -> [_ _ _ _ _ _ _ w5358 _ _]
                          tunnel: [_ _ _ _ _ _ _ w5357 _ _] -> w5267
                          tunnel: w5266 -> [_ _ _ _ _ _ _ _ w5368 _]
                          tunnel: [_ _ _ _ _ _ _ _ w5367 _] -> w5265
                          tunnel: w5264 -> [_ _ _ _ _ _ _ _ _ w5378]
                          tunnel: [_ _ _ _ _ _ _ _ _ w5377] -> w5263
                          frame #0 {
                            n2849 = Greater?(x=w5288, y=w5291) -> (0:w5290:bool)
                            n2850 = case shown="True" w5290 {
                              tunnel: [w5292 0] -> w5289
                              tunnel: w5288 -> [w5292 _]
                              tunnel: w5287 -> [_ w5293]
                              frame False {
                              }
                              frame True {
                                n2851 = Concatenate Strings("LA01-1 ", w5293) -> (w5296:string)
                                n2852 = One Button Dialog(message=w5296) -> ()  [unwired: 1 in, 1 out]
                              }
                            }
                          }
                          frame #1 {
                            n2853 = Greater?(x=w5297, y=w5301) -> (0:w5300:bool)
                            n2854 = case shown="True" w5300 {
                              tunnel: [w5302 0] -> w5298
                              tunnel: w5297 -> [w5302 _]
                              tunnel: w5299 -> [_ w5303]
                              frame False {
                              }
                              frame True {
                                n2855 = Concatenate Strings("LA01-2 ", w5303) -> (w5306:string)
                                n2856 = One Button Dialog(message=w5306) -> ()  [unwired: 1 in, 1 out]
                              }
                            }
                          }
                          frame #2 {
                            n2857 = Greater?(x=w5307, y=w5311) -> (0:w5310:bool)
                            n2858 = case shown="True" w5310 {
                              tunnel: [w5312 0] -> w5308
                              tunnel: w5307 -> [w5312 _]
                              tunnel: w5309 -> [_ w5313]
                              frame False {
                              }
                              frame True {
                                n2859 = Concatenate Strings("LA02-1 ", w5313) -> (w5316:string)
                                n2860 = One Button Dialog(message=w5316) -> ()  [unwired: 1 in, 1 out]
                              }
                            }
                          }
                          frame #3 {
                            n2861 = Greater?(x=w5318, y=w5321) -> (0:w5320:bool)
                            n2862 = case shown="True" w5320 {
                              tunnel: [w5322 0] -> w5317
                              tunnel: w5318 -> [w5322 _]
                              tunnel: w5319 -> [_ w5323]
                              frame False {
                              }
                              frame True {
                                n2863 = Concatenate Strings("LA02-2 ", w5323) -> (w5326:string)
                                n2864 = One Button Dialog(message=w5326) -> ()  [unwired: 1 in, 1 out]
                              }
                            }
                          }
                          frame #4 {
                            n2865 = Greater?(x=w5328, y=w5331) -> (0:w5330:bool)
                            n2866 = case shown="True" w5330 {
                              tunnel: [w5332 0] -> w5327
                              tunnel: w5328 -> [w5332 _]
                              tunnel: w5329 -> [_ w5333]
                              frame False {
                              }
                              frame True {
                                n2867 = Concatenate Strings("LA03-1 ", w5333) -> (w5336:string)
                                n2868 = One Button Dialog(message=w5336) -> ()  [unwired: 1 in, 1 out]
                              }
                            }
                          }
                          frame #5 {
                            n2869 = Greater?(x=w5337, y=w5341) -> (0:w5340:bool)
                            n2870 = case shown="True" w5340 {
                              tunnel: [w5342 0] -> w5338
                              tunnel: w5337 -> [w5342 _]
                              tunnel: w5339 -> [_ w5343]
                              frame False {
                              }
                              frame True {
                                n2871 = Concatenate Strings("LA03-2 ", w5343) -> (w5346:string)
                                n2872 = One Button Dialog(message=w5346) -> ()  [unwired: 1 in, 1 out]
                              }
                            }
                          }
                          frame #6 {
                            n2873 = Greater?(x=w5348, y=w5351) -> (0:w5350:bool)
                            n2874 = case shown="True" w5350 {
                              tunnel: [w5352 0] -> w5347
                              tunnel: w5348 -> [w5352 _]
                              tunnel: w5349 -> [_ w5353]
                              frame False {
                              }
                              frame True {
                                n2875 = Concatenate Strings("LA04-1 ", w5353) -> (w5356:string)
                                n2876 = One Button Dialog(message=w5356) -> ()  [unwired: 1 in, 1 out]
                              }
                            }
                          }
                          frame #7 {
                            n2877 = Greater?(x=w5358, y=w5361) -> (0:w5360:bool)
                            n2878 = case shown="True" w5360 {
                              tunnel: [w5362 0] -> w5357
                              tunnel: w5358 -> [w5362 _]
                              tunnel: w5359 -> [_ w5363]
                              frame False {
                              }
                              frame True {
                                n2879 = Concatenate Strings("LA04-2 ", w5363) -> (w5366:string)
                                n2880 = One Button Dialog(message=w5366) -> ()  [unwired: 1 in, 1 out]
                              }
                            }
                          }
                          frame #8 {
                            n2881 = Greater?(x=w5368, y=w5371) -> (0:w5370:bool)
                            n2882 = case shown="True" w5370 {
                              tunnel: [w5372 0] -> w5367
                              tunnel: w5368 -> [w5372 _]
                              tunnel: w5369 -> [_ w5373]
                              frame False {
                              }
                              frame True {
                                n2883 = Concatenate Strings("LA05-1 ", w5373) -> (w5376:string)
                                n2884 = One Button Dialog(message=w5376) -> ()  [unwired: 1 in, 1 out]
                              }
                            }
